vi "Write Weights.vi"(8 "error in (no error)":errorcluster, 10 "Weights":T1=enum."Pink", 11 "Noise in":refnum<class "Noise.lvclass">) -> (0 "error out":errorcluster, 3 "Noise out":refnum<class "Noise.lvclass">)   [LabVIEW 2020, in "Noise.lvclass"]
uses:
  Noise.lvclass
  Weighting.ctl
  Noise.lvclass/Noise.ctl
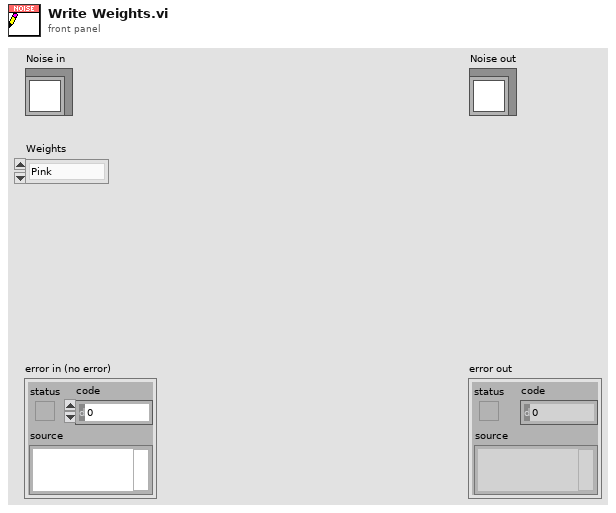
[diagram p1: front panel]
types:
  T1 = typedef "Noise.lvclass/Weighting.ctl" = enum16{"White", "Pink"}
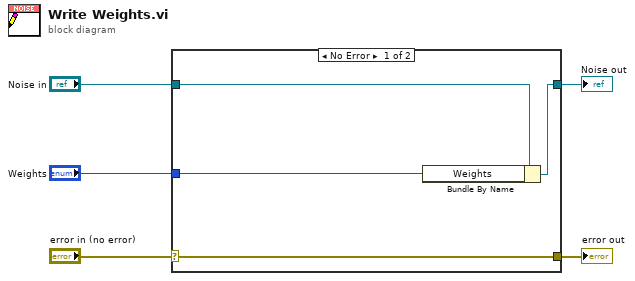
[diagram p0: block diagram]
diagram:
  n1 = case shown="No Error" "error in (no error)" {
    selector: "error in (no error)" -> [w9 w10]
    tunnel: [w9 w10] -> w4
    tunnel: [w7 w11] -> w2
    tunnel: "Noise in" -> [w8 w11]
    tunnel: "Weights" -> [w6 _]
    frame No Error {
      n2 = Bundle By Name(cluster=w8, "Weights"=w6) -> (w7:refnum<class "Noise.lvclass">)
    }
    frame Error {
    }
  }
  "error out" <- w4
  "Noise out" <- w2
